vi "GDSString_ParseBaseMethodCall.vi"(4 "TextInsideParenthesesForBaseMethodCall":string, 9 "TextBeforeBlock":string, 10 "IndexOfStartOfBaseParentheses":i32) -> (1 "MethodArgumentsString":string, 2 "IndexBeforeReturnTypeMatch":i32, 3 "Word2(method Return Type)":string, 5 "Word1(Method name)":string)   [LabVIEW 2016]
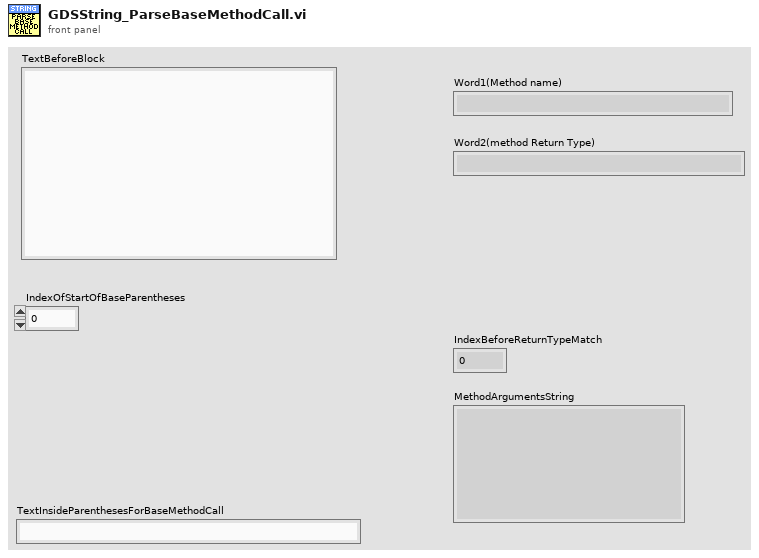
[diagram p1: front panel]
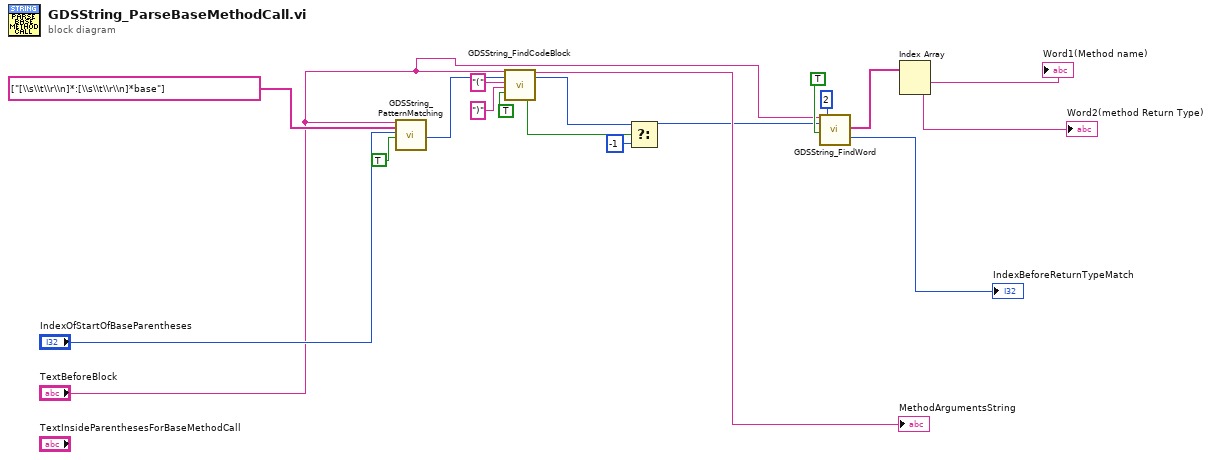
[diagram p0: block diagram]
diagram:
  n1 = call <resource>:"GDSString_PatternMatching.vi"("TextIn"="TextBeforeBlock", "PatternMatchingStrings"=string[] ["[\\s\\t\\r\\n]*:[\\s\\t\\r\\n]*base"], "StringStartOffset(Default=-1 => 0 for Forward, StrLenght for Backwards)"="IndexOfStartOfBaseParentheses", "Search Backwards"=TRUE) -> ("IndexAfterMatch(Or before when searching Backwards)"=w13:i32)  [unwired: 9 in, 6 out]
  n2 = call <resource>:"GDSString_FindCodeBlock.vi"("Text"="TextBeforeBlock", "StringStartOffset(Default=-1 => 0 for Forward, StrLenght for Backwards)"=w13, "CodeBlockStartCharacter( { )"="(", "CodeBlockEndCharacter( } )"=")", "Search Backwards"=TRUE) -> ("found"=w10:bool, "BlockText"=→"MethodArgumentsString":string, "BlockStart(Outside)"=w9:i32)  [unwired: 6 in, 6 out]
  n3 = Select(t=w9, s=w10, f=-1) -> (s? t:f=w6:i32)
  n4 = call <resource>:"GDSString_FindWord.vi"("Text"="TextBeforeBlock", "StringStartOffset(Default=-1 => 0 for Forward, StrLenght for Backwards)"=w6, "Search Backwards"=TRUE, "GetNext-X_Words(1,-1=All)"=2 ("GetNext-X_Words(1)")) -> ("NextWords"=w4:string[], "IndexAfterLastMatch(Or before when searching Backwards)"=→"IndexBeforeReturnTypeMatch":i32)  [unwired: 10 in, 4 out]
  n5 = Index Array(array=w4) -> (element #1=→"Word1(Method name)":string, element #2=→"Word2(method Return Type)":string)  [unwired: 2 in]
